vi "Destroy.vi"(8 "error in (no error)":errorcluster, 11 "Subroutine in":refnum<class "Subroutine.lvclass">) -> (0 "error out":errorcluster)   [LabVIEW 2019, in "Test Executive.lvlib" / "Subroutine.lvclass"]
uses:
  <vilib>/gpm_packages/@cs/test-executive/Source/Test Executive/Subroutine/Subroutine.lvclass
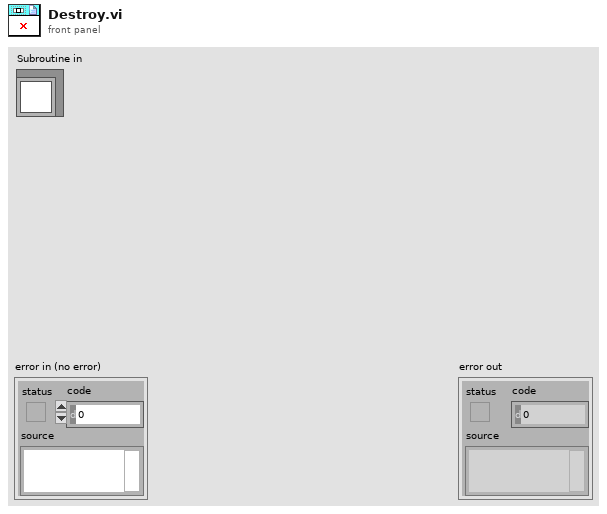
[diagram p1: front panel]
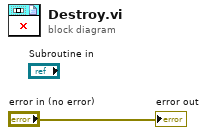
[diagram p0: block diagram]
diagram:
  "error out" <- "error in (no error)"
